vi "Test22.vi"() -> ()   [LabVIEW 2019]
panel:
  in  "CameraName":string="cam01"
  in  "Index":i32
  in  "Load File Path":string="C:\\Users\\Public\\Documents\\National Instruments\\Vision\\Examples\\Images\\Battery\\Image00.jpg"
  in  "Load Template":bool
  in  "coordinate space":bool
  in  "Run":bool
  in  "Enabled/Disabled":bool
  in  "script path":string="C:\\Users\\chenju\\Desktop\\iVision_20160423_Caliper_Coor -Cal\\Data\\123"
  in  "stop":bool
  out "data string":string
  # "<- Run之前要改"
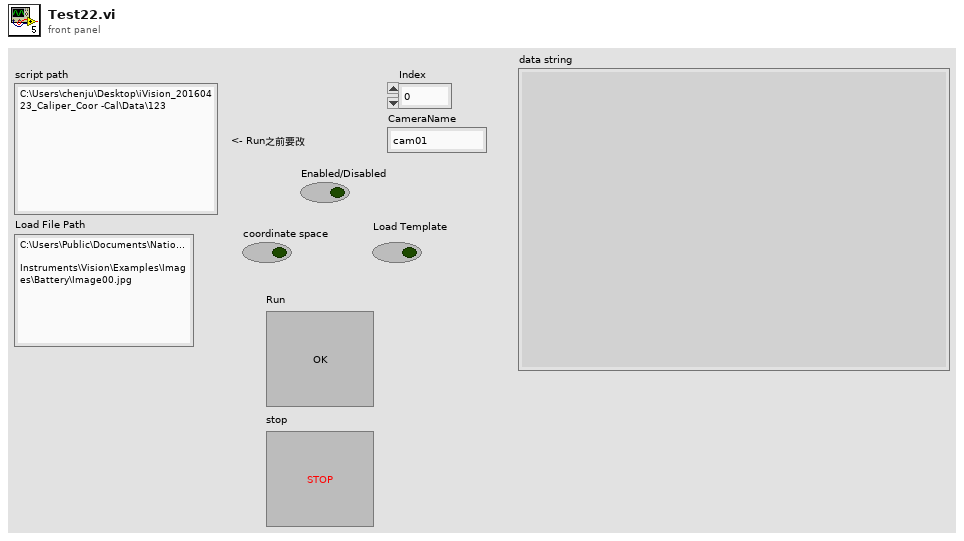
[diagram p1: front panel]
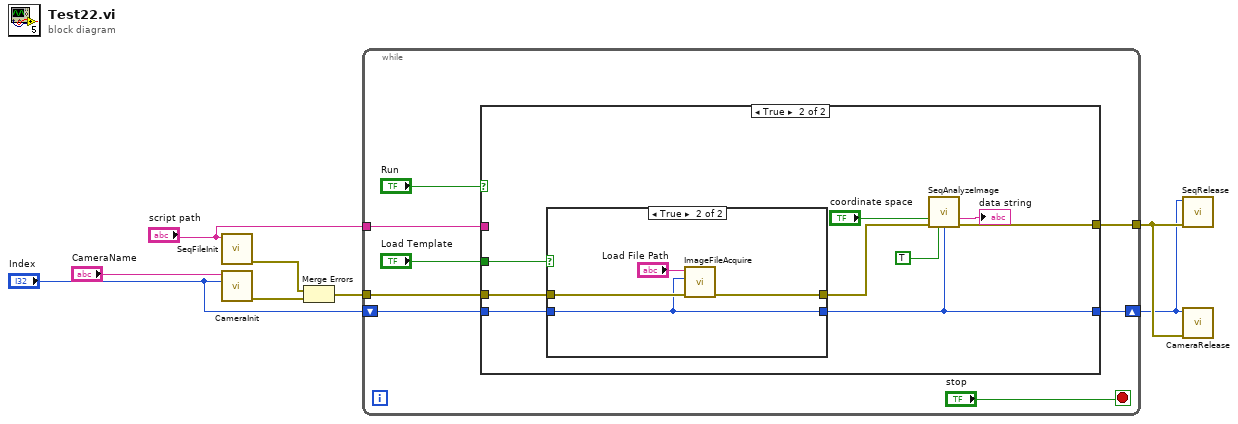
[diagram p0: block diagram]
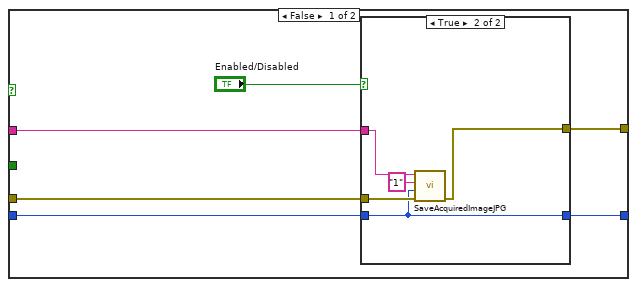
[diagram p2: hidden frame]
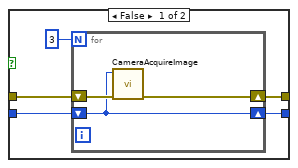
[diagram p4: hidden frame]
diagram:
  n1 = call "SeqFileInit.vi"("script path"="script path") -> ("error out"=w6:errorcluster)  [unwired: 9 in, 1 out]
  n2 = call "CameraInit.vi"("Index"="Index", "CameraName"="CameraName") -> ("error out"=w8:errorcluster)  [unwired: 8 in, 1 out]
  n3 = Merge Errors(w6, w8) -> (w7:errorcluster)
  n4 = while {
    tunnel: w7 -> [w15]
    tunnel: [w14] -> w5
    tunnel: "script path" -> [w13]
    shift-right: [w9] -> w1
    shift-left: "Index" -> [w10]
    stop <- "stop" stop-if-true
    n5 = case shown="True" "Run" {
      tunnel: w15 -> [w21 w38]
      tunnel: [w20 w36] -> w14
      tunnel: w13 -> [w19 _]
      tunnel: "Load Template" -> [_ w33]
      tunnel: w10 -> [w18 w32]
      tunnel: [w17 w30] -> w9
      frame False {
        n6 = case shown="True" "Enabled/Disabled" {
          tunnel: w21 -> [w24 w29]
          tunnel: [w24 w28] -> w20
          tunnel: w19 -> [_ w27]
          tunnel: w18 -> [w23 w25]
          tunnel: [w23 w25] -> w17
          frame False {
          }
          frame True {
            n7 = call "SaveAcquiredImageJPG.vi"("error in"=w29, "Index"=w25, "File Name"="1", "Folder Path"=w27) -> ("error out"=w28:errorcluster)  [unwired: 4 in, 3 out]
          }
        }
      }
      frame True {
        n8 = case shown="True" w33 {
          tunnel: w38 -> [w43 w50]
          tunnel: [w42 w49] -> w37
          tunnel: w32 -> [w40 w47]
          tunnel: [w39 w47] -> w30
          frame False {
            n9 = for {
              N: 3 -> [_]
              shift-right: [w45] -> w42
              shift-left: w43 -> [w46]
              shift-right: [w44] -> w39
              shift-left: w40 -> [w44]
              n10 = call "CameraAcquireImage.vi"("error in"=w46, "Index"=w44) -> ("error out"=w45:errorcluster)  [unwired: 8 in, 1 out]
            }
          }
          frame True {
            n11 = call "ImageFileAcquire.vi"("error in"=w50, "Index"=w47, "File Path"="Load File Path") -> ("error out"=w49:errorcluster)  [unwired: 7 in, 1 out]
          }
        }
        n12 = call "SeqAnalyzeImage.vi"("coordinate space"="coordinate space", "error in"=w37, "CreatDllImage"=TRUE, "Cam Index"=w30) -> ("data string"=→"data string":string, "error out"=w36:errorcluster)  [unwired: 6 in, 4 out]
      }
    }
  }
  n13 = call "SeqRelease.vi"("error in"=w5, "Index"=w1) -> ()  [unwired: 8 in, 2 out]
  n14 = call "CameraRelease.vi"("error in"=w5, "Index"=w1) -> ()  [unwired: 8 in, 2 out]
